vi "Configure movement.vi"(7 "Final wavelength":dbl, 8 "error in (no error)":errorcluster, 9 "Initial wavelength":dbl, 10 "Mono Mod ID":i32, 11 "Speed":dbl) -> (0 "error out":errorcluster)   [LabVIEW 2020]
uses:
  Monochromator/Libraries/Monochromator/Monochromator.lvlib
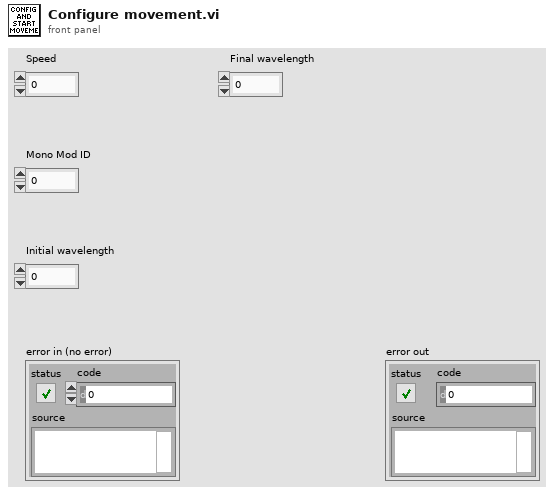
[diagram p1: front panel]
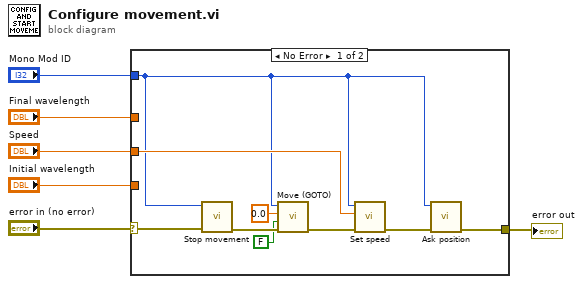
[diagram p0: block diagram]
diagram:
  n1 = case shown="No Error" "error in (no error)" {
    selector: "error in (no error)" -> [w12 w16]
    tunnel: "Initial wavelength" -> [_ _]
    tunnel: "Mono Mod ID" -> [w8 _]
    tunnel: [w9 w16] -> w4
    tunnel: "Speed" -> [w13 _]
    tunnel: "Final wavelength" -> [_ _]
    frame No Error {
      n2 = call "Stop movement.vi"("error in"=w12, "Module ID"=w8) -> ("error out"=w14:errorcluster)  [unwired: 9 in]
      n3 = call "Move (GOTO).vi"("error in"=w14, "Echo?"=FALSE, "Position"=0.0, "Module ID"=w8) -> ("error out"=w15:errorcluster)  [unwired: 6 in, 1 out]
      n4 = call "Set speed.vi"("error in"=w15, "nm/min"=w13, "Module ID"=w8) -> ("error out"=w10:errorcluster)  [unwired: 8 in]
      n5 = call "Ask position.vi"("error in"=w10, "Module ID"=w8) -> ("error out"=w9:errorcluster)  [unwired: 7 in, 2 out]
    }
    frame Error {
    }
  }
  "error out" <- w4
